vi "Export Clock.vi"(0 "device session in":refnum<class "Device Session.lvclass">, 5 "exported clock":T2, 7 "output terminal":T1="Do Not Export", 11 "error in":errorcluster) -> (4 "device session out":refnum<class "Device Session.lvclass">, 15 "error out":errorcluster)   [LabVIEW 2021, in "Device Session.lvclass"]
doc: "Exports the ADC clock signal or reference clock signal to a specified output terminal. If the clock to export has not been configured, this VI will return an error.\n\n<B>Input Parameters</B>\n\n<B>device session in</B> is a reference to the Device Session object, which contains a session to each instrument design library used in this sample project. This parameter is obtained from the 'Open Session' VI.\n\n<B>exported clock</B> specifies the clock signal to export.\n\n'None': No clock signal will be exported.\n'ADC Clock': The ADC clock signal will be exported.\n'PLL Reference Clock': The phase-locked reference clock signal will be exported.\n\n<B>output terminal</B> specifies the terminal to which the clock signal will be exported. You can choose not to export any signal.\n'Do Not Export': Specifies that the signal is not exported.\n'Clock Out': Specifies that the signal is exported to the CLK OUT terminal.\n\n<B>error in</B> describes error conditions that occur before this node runs. This input provides standard 'error in' functionality.\n\n<B>Output Parameters</B>\n\n<B>device session out</B> passes a reference to the session to the next VI.\n\n<B>error out</B> contains error information. This output provides standard 'error out' functionality."
uses:
  Device Session.lvclass
  <instrlib>/HSAI-RIO/Types/v1/Host/Typedefs/Exported Clock.ctl
  <instrlib>/HSAI-RIO/Types/v1/Host/Typedefs/output terminal.ctl
  Device Session.lvclass/Device Session.ctl
  <instrlib>/HSAI-RIO/Config/Group A/v1/Host/Main/niHSAI Group A Config v1 Host.lvclass
  <instrlib>/HSAI-RIO/Types/v1/Host/niHSAI Types v1 Host.lvlib
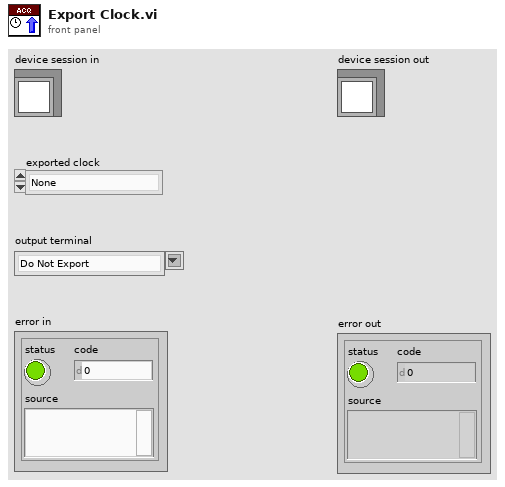
[diagram p1: front panel]
types:
  T1 = typedef "niHSAI Types v1 Host.lvlib/output terminal.ctl" = string
  T2 = typedef "niHSAI Types v1 Host.lvlib/Exported Clock.ctl" = enum8{"None", "ADC Clock", "PLL Reference Clock"}
  T3 = typedef "Device Session.lvclass/Device Session Object.ctl" = cluster{"fpga reference":T4, "reg bus":refnum<class "niInstr FIFO Register Bus v1 Host.lvclass">, "subsystem map":refnum<class "niInstr Subsystem Map v1 Host.lvclass">, "cal data":refnum<class "niHSAI Cal Data v1 Host.lvclass">, "config":refnum<class "niHSAI Group A Config v1 Host.lvclass">, "acquisition":refnum<class "niInstr Multirecord Acquisition v1 Host.lvclass">, "number of selected acq channels":u8, "selected acq channels":bool[], "number of channels":u32, "configured channels":bool[], "acq configuration":cluster{"number of samples":u64, "number of records":u64, "pretrigger samples":u64}, "actual channel configuration":T5[], "sample clock rate (Hz)":dbl, "scaling coefficients":T9[]}
  T4 = typedef "Device Session.lvclass/FPGA Refnum.ctl" = refnum<k20>
  T5 = typedef "niHSAI Types v1 Host.lvlib/Channel Configuration.ctl" = cluster{"channel":u32, "coupling":T6, "impedance":T7, "bandwidth":T8, "vertical range":dbl, "vertical offset":dbl}
  T6 = typedef "niHSAI Types v1 Host.lvlib/Coupling.ctl" = enum8{"Default", "DC", "AC"}
  T7 = typedef "niHSAI Types v1 Host.lvlib/Impedance.ctl" = enum8{"Default", "1 mega ohm", "50 ohm"}
  T8 = typedef "niHSAI Types v1 Host.lvlib/Bandwidth.ctl" = enum8{"Default", "Full Bandwidth", "Anti-alias Filter", "150 MHz"}
  T9 = typedef "niInstr Multirecord Acquisition v1 Host.lvclass/Scaling Coefficient.ctl" = cluster{"gain":dbl, "offset":dbl}
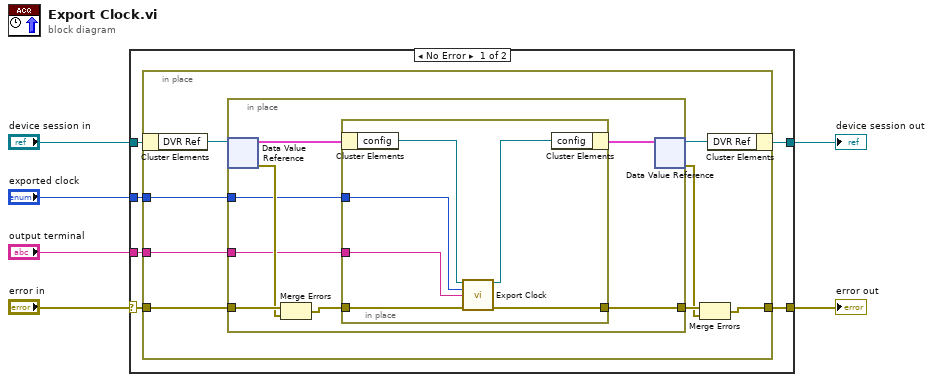
[diagram p0: block diagram]
diagram:
  n1 = case shown="No Error" "error in" {
    selector: "error in" -> [w12 w36]
    tunnel: "device session in" -> [w8 w35]
    tunnel: [w7 w35] -> w4
    tunnel: [w11 w36] -> w3
    tunnel: "exported clock" -> [w10 _]
    tunnel: "output terminal" -> [w9 _]
    frame No Error {
      n2 = in-place {
        in-place-border: w12 -> [w20]
        in-place-border: [w18] -> w11
        in-place-border: w10 -> [w16]
        in-place-border: w9 -> [w15]
        n3 = in-place-cluster #1(w8) -> ("DVR Ref"=w14:refnum<data-value>)
        n4 = in-place {
          in-place-border: w20 -> [w27]
          in-place-border: [w28] -> w19
          in-place-border: w16 -> [w22]
          in-place-border: w15 -> [w23]
          n5 = in-place-dvr #2(w14) -> (w24:T3, w26:errorcluster)
          n6 = Merge Errors(w27, w26) -> (w25:errorcluster)
          n7 = in-place {
            in-place-border: [w34] -> w28
            in-place-border: w25 -> [w33]
            in-place-border: w23 -> [w32]
            in-place-border: w22 -> [w31]
            n8 = in-place-cluster #3(w24) -> ("config"=w30:refnum<class "niHSAI Group A Config v1 Host.lvclass">)
            n9 = call-dynamic "Export Clock.vi"("session in"=w30, "exported clock"=w31, "output terminal"=w32, "error in"=w33) -> ("session out"=w29:refnum<class "niHSAI Group A Config v1 Host.lvclass">, "error out"=w34:errorcluster)  [unwired: 10 in]
            n10 = in-place-cluster #3("config"=w29) -> (w21:T3)
          }
          n11 = in-place-dvr #2(w21) -> (w13:refnum<data-value>, w17:errorcluster)
        }
        n12 = Merge Errors(w19, w17) -> (w18:errorcluster)
        n13 = in-place-cluster #1("DVR Ref"=w13) -> (w7:refnum<class "Device Session.lvclass">)
      }
    }
    frame Error {
    }
  }
  "error out" <- w3
  "device session out" <- w4
